vi "Begin.vi"(8 "error in (no error)":errorcluster, 9 "Pneumatics control.lvlib:Solenoids.lvclass":refnum<class "Solenoids.lvclass">, 10 "Settings":variant, 11 "Pneumatics in":refnum<class "Pneumatics.lvclass">) -> (0 "error out":errorcluster, 3 "Pneumatics out":refnum<class "Pneumatics.lvclass">)   [LabVIEW 2019, in "Pneumatics control.lvlib" / "Pneumatics.lvclass"]
doc: "This VI instantiates the solenoids in the pnaumatic class, and sets both the channels and the PCM id based on the configuration input we receive."
uses:
  Pneumatics.lvclass
  Solenoids/Solenoids.lvclass
  TypeDefs/Solenoids.ctl
  Pneumatics.lvclass/Pneumatics.ctl
  df110fe4-3670-4473-9499-9f180371a8d4.vi
  <vilib>/Utility/error.llb/Trim Whitespace.vi
  <vilib>/Utility/error.llb/Error Cluster From Error Code.vi
  <vilib>/Rock Robotics/WPI/Utilities/WPI_GetSetVariantRefNum.vi
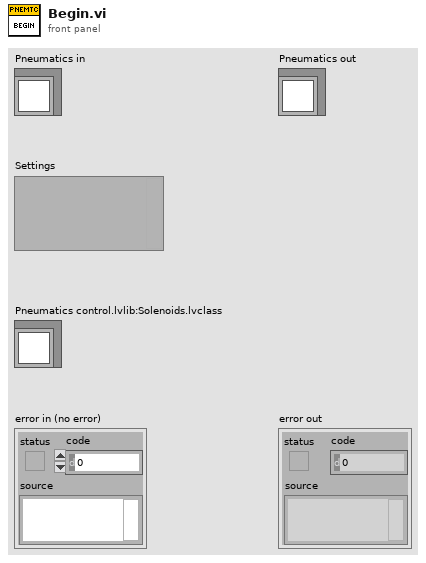
[diagram p1: front panel]
types:
  T1 = typedef "Pneumatics control.lvlib/Pneumatics.lvclass/Solenoids.ctl" = cluster{"Air Cooler":refnum<class "Solenoids.lvclass">, "ArmLock":refnum<class "Solenoids.lvclass">, "HatchArm":refnum<class "Solenoids.lvclass">, "HatchGrabber":refnum<class "Solenoids.lvclass">, "CPDeploy":refnum<class "Solenoids.lvclass">, "Power Cells Intake":refnum<class "Solenoids.lvclass">}
  T2 = typedef "WPI_CompressorDevRef.ctl" = cluster{"DevStatus":errorcluster, "Pneumatics Control Module":u8}
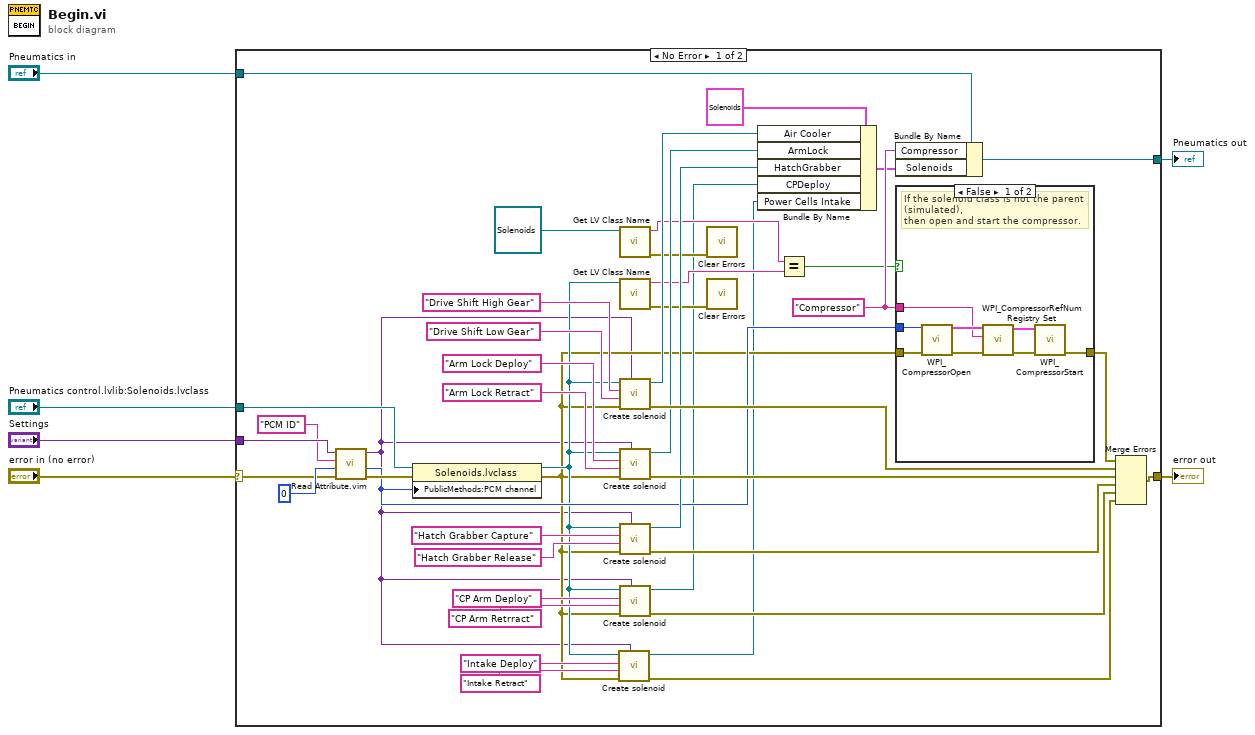
[diagram p0: block diagram]
diagram:
  n1 = case shown="No Error" "error in (no error)" {
    selector: "error in (no error)" -> [w42 w60]
    tunnel: [w38 w60] -> w5
    tunnel: [w48 w59] -> w3
    tunnel: "Pneumatics in" -> [w49 w59]
    tunnel: "Settings" -> [w45 _]
    tunnel: "Pneumatics control.lvlib:Solenoids.lvclass" -> [w19 _]
    frame No Error {
      w47 = "Compressor" ("refnum name")
      n2 = call "Read Attribute.vim"("error in"=w42, "default value (data type)"=u8 0, "name"="PCM ID", "variant in"=w45) -> ("error out"=w36:errorcluster, "value"=w18:u8, "variant out"=w9:variant)  [unwired: 4 in, 1 out]
      n3 = property class="Solenoids.lvclass"(reference=w19, error in=w36, "PublicMethods:PCM channel"=w18) -> (reference out=w11:refnum<class "Solenoids.lvclass">, error out=w10:errorcluster)
      n4 = call "Create solenoid.vi"("Variant"=w9, "error in (no error)"=w10, "Reverse solenoid channel"="Intake Retract", "Forward solenoid channel"="Intake Deploy", "Solenoids in"=w11) -> ("error out"=w7:errorcluster, "Solenoids out"=w8:refnum<class "Solenoids.lvclass">)  [unwired: 5 in]
      n5 = call <vilib>:"Get LV Class Name.vi"("object"=refnum<class "Solenoids.lvclass"> refnum ("Pneumatics control.lvlib:Solenoids.lvclass")) -> ("error out"=w21:errorcluster, "class name"=w24:string)  [unwired: 9 in]
      n6 = call <vilib>:"Get LV Class Name.vi"("object"=w11) -> ("error out"=w20:errorcluster, "class name"=w23:string)  [unwired: 9 in]
      n7 = call "Create solenoid.vi"("Variant"=w9, "error in (no error)"=w10, "Reverse solenoid channel"="Drive Shift Low Gear", "Forward solenoid channel"="Drive Shift High Gear", "Solenoids in"=w11) -> ("error out"=w37:errorcluster, "Solenoids out"=w39:refnum<class "Solenoids.lvclass">)  [unwired: 5 in]
      n8 = call "Create solenoid.vi"("Variant"=w9, "error in (no error)"=w10, "Reverse solenoid channel"="Arm Lock Retract", "Forward solenoid channel"="Arm Lock Deploy", "Solenoids in"=w11) -> ("error out"=w34:errorcluster, "Solenoids out"=w32:refnum<class "Solenoids.lvclass">)  [unwired: 5 in]
      n9 = call "Create solenoid.vi"("Variant"=w9, "error in (no error)"=w10, "Reverse solenoid channel"="Hatch Grabber Release", "Forward solenoid channel"="Hatch Grabber Capture", "Solenoids in"=w11) -> ("error out"=w35:errorcluster, "Solenoids out"=w33:refnum<class "Solenoids.lvclass">)  [unwired: 5 in]
      n10 = call "Create solenoid.vi"("Variant"=w9, "error in (no error)"=w10, "Reverse solenoid channel"="CP Arm Retrract", "Forward solenoid channel"="CP Arm Deploy", "Solenoids in"=w11) -> ("error out"=w15:errorcluster, "Solenoids out"=w14:refnum<class "Solenoids.lvclass">)  [unwired: 5 in]
      n11 = call <vilib>:"Clear Errors.vi"("error in (no error)"=w21) -> ()  [unwired: 5 in, 2 out]
      n12 = call <vilib>:"Clear Errors.vi"("error in (no error)"=w20) -> ()  [unwired: 5 in, 2 out]
      n13 = Bundle By Name(cluster=T1 {"Air Cooler"=refnum, "ArmLock"=refnum, "HatchArm"=refnum, "HatchGrabber"=refnum, "CPDeploy"=refnum, "Power Cells Intake"=refnum} ("Solenoids"), "Air Cooler"=w39, "ArmLock"=w32, "HatchGrabber"=w33, "CPDeploy"=w14, "Power Cells Intake"=w8) -> (w40:T1)
      n14 = Equal?(x=w24, y=w23) -> (x = y?=w22:bool)
      n15 = Bundle By Name(cluster=w49, "Compressor"=w47, "Solenoids"=w40) -> (w48:refnum<class "Pneumatics.lvclass">)
      n16 = case shown="False" w22 {
        tunnel: w47 -> [w53 _]
        tunnel: [w52 w58] -> w46
        tunnel: w10 -> [w51 w58]
        tunnel: w18 -> [w50 _]
        frame False {
          # "If the solenoid class is not the parent (simulated),\nthen open and start the compressor."
          n17 = call <vilib>:"WPI_CompressorOpen.vi"("Pneumatics Control Module (0)"=w50, "error in (no error)"=w51) -> ("CompressorDevRef"=w57:T2, "error out"=w55:errorcluster)  [unwired: 12 in]
          n18 = call <vilib>:"WPI_CompressorRefNum Registry Set.vi"("error in (no error)"=w55, "refnum name"=w53, "CompressorDevRef"=w57) -> ("error out"=w54:errorcluster, "CompressorDevRef"=w56:T2)  [unwired: 7 in]
          n19 = call <vilib>:"WPI_CompressorStart.vi"("error in (no error)"=w54, "CompressorDevRef"=w56) -> ("error out"=w52:errorcluster)  [unwired: 8 in, 1 out]
        }
        frame True {
          # "If simulated, then do not open the compressor"
        }
      }
      n20 = Merge Errors(w46, w37, w34, w35, w15, w7) -> (w38:errorcluster)
    }
    frame Error {
    }
  }
  "error out" <- w5
  "Pneumatics out" <- w3
